vi "Array Subset.vi"(0 "JSON Value in":refnum<class "JSON Value.lvclass">, 7 "index":i32, 9 "length":i32, 11 "error in (no error)":errorcluster) -> (8 "JSON Value out":refnum<class "JSON Value.lvclass">, 15 "error out":errorcluster)   [LabVIEW 2016, in "JSON Value.lvclass"]
doc: "Returns a subset of a JSON Array"
uses:
  JSON Value.lvclass
  New JSON Value/New JSON (Value[]).vi
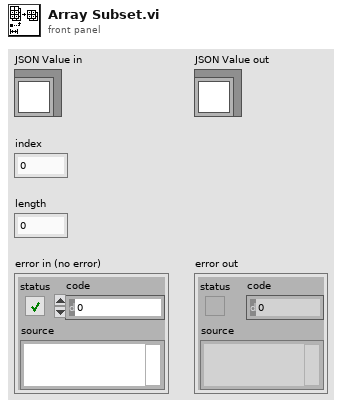
[diagram p1: front panel]
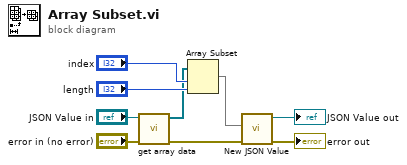
[diagram p0: block diagram]
diagram:
  n1 = call "get array data.vi"("error in (no error)"="error in (no error)", "JSON Value in"="JSON Value in") -> ("error out"=w3:errorcluster, "JSON Array out"=w5:refnum<class "JSON Value.lvclass">[])  [unwired: 8 in]
  n2 = Array Subset(array=w5, index="index", length="length") -> (w7:refnum<class "JSON Value.lvclass">[])
  n3 = call-poly "New JSON Value.vi"("error in (no error)"=w3, "JSON Datatypes"=w7) -> ("error out"=→"error out":errorcluster, "JSON Value out"=→"JSON Value out":refnum<class "JSON Value.lvclass">)  [unwired: 8 in]
